vi "Execute.vi"(6 "WhereIGetMyInformationDescription":string, 8 "error in (no error)":errorcluster caption="Fehler (Eingang, kein Fehler)", 9 "WhereIGetMyInformationLocation":string, 10 "WhoIAm":string, 11 "ApllicationLoadAndConfigurationFileBasedClass Eingang":refnum<class "LoadConfigurationFileBasedClass.lvclass"> caption="DNL_LabVIEW Object in") -> (0 "error out":errorcluster caption="Fehler (Ausgang)", 2 "LvDictionary.lvlib:DictionaryString.lvclass":refnum<class "DictionaryString.lvclass">, 3 "ApllicationLoadAndConfigurationFileBasedClass Ausgang":refnum<class "LoadConfigurationFileBasedClass.lvclass"> caption="DNL_LabVIEW Object out")   [LabVIEW 2013, in "LoadConfigurationFileBasedClass.lvclass"]
uses:
  LoadConfigurationFileBasedClass.lvclass
  LvDictionary/DictionaryStringClass/DictionaryString.lvclass
  <vilib>/Utility/config.llb/Read Key (String).vi
  <vilib>/Utility/config.llb/NI_LVConfig.lvlib
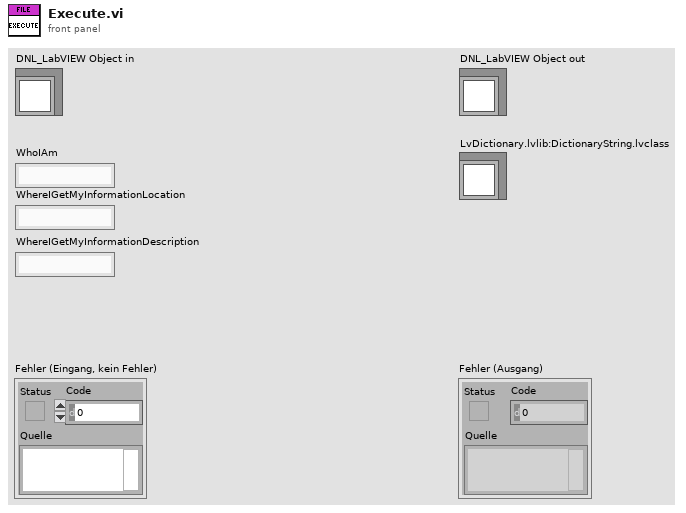
[diagram p1: front panel]
types:
  T1 = typedef "NI_LVConfig.lvlib/Config Data RefNum.ctl" = refnum<k1>
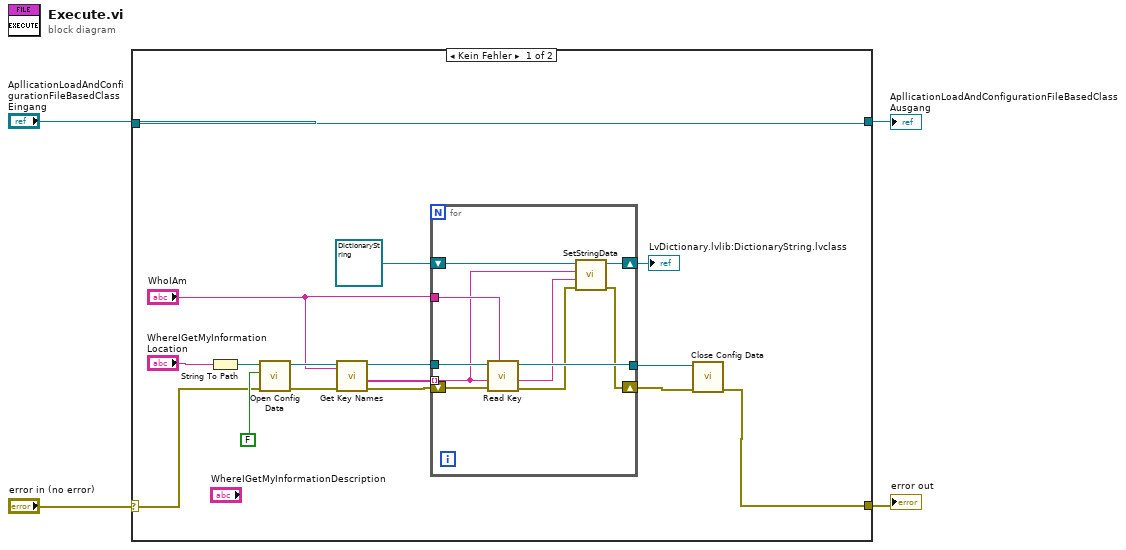
[diagram p0: block diagram]
diagram:
  n1 = case shown="Kein Fehler" "error in (no error)" {
    selector: "error in (no error)" -> [w12 w32]
    tunnel: [w9 w32] -> w4
    tunnel: "ApllicationLoadAndConfigurationFileBasedClass Eingang" -> [w20 w31]
    tunnel: [w20 w31] -> w2
    frame No Error {
      n2 = String To Path(string="WhereIGetMyInformationLocation") -> (path=w16:path)
      n3 = call <vilib>:"Open Config Data.vi"("error in (no error)"=w12, "create file if necessary (T)"=FALSE, "configuration file path"=w16) -> ("error out"=w19:errorcluster, "refnum"=w15:T1)  [unwired: 6 in, 1 out]
      n4 = call <vilib>:"Get Key Names.vi"("section"="WhoIAm", "error in (no error)"=w19, "refnum"=w15) -> ("error out"=w11:errorcluster, "key names"=w14:string[], "refnum out"=w13:T1)  [unwired: 5 in, 1 out]
      n5 = for {
        tunnel: w14 -> [w25] mode=indexing
        tunnel: w13 -> [w30]
        shift-right: [w22] -> w10
        shift-left: w11 -> [w29]
        tunnel: [w28] -> w8
        tunnel: "WhoIAm" -> [w27]
        shift-right: [w21] -> w6
        shift-left: refnum<class "DictionaryString.lvclass"> refnum ("LvDictionary.lvlib:DictionaryString.lvclass") -> [w26]
        n6 = call-poly <vilib>:"Read Key.vi"("section"=w27, "error in (no error)"=w29, "key"=w25, "refnum"=w30) -> ("error out"=w23:errorcluster, "value"=w24:string, "refnum out"=w28:T1)  [unwired: 4 in, 1 out]
        n7 = call-dynamic "SetStringData.vi"("error in (no error)"=w23, "Value"=w24, "Name"=w25, "DictionaryString Eingang"=w26) -> ("error out"=w22:errorcluster, "DictionaryString Ausgang"=w21:refnum<class "DictionaryString.lvclass">)  [unwired: 6 in]
      }
      "LvDictionary.lvlib:DictionaryString.lvclass" <- w6
      n8 = call <vilib>:"Close Config Data.vi"("error in (no error)"=w10, "refnum"=w8) -> ("error out"=w9:errorcluster)  [unwired: 8 in, 1 out]
    }
    frame Error {
    }
  }
  "error out" <- w4
  "ApllicationLoadAndConfigurationFileBasedClass Ausgang" <- w2
